vi "_power value.vi"(6 "label":T1, 8 "error in (no error)":errorcluster, 10 "B":refnum<class "Value.lvclass">, 11 "A":refnum<class "Value.lvclass">) -> (0 "error out":errorcluster, 2 "C":refnum<class "Value.lvclass">, 3 "A out":refnum<class "Value.lvclass">)   [LabVIEW 2023, in "LabGRAD.lvlib" / "Value.lvclass"]
uses:
  Value.lvclass
  UiObjects/string control.ctl
  operation.ctl
  Value.lvclass/Value.ctl
  UiObjects/UiObjects.lvclass
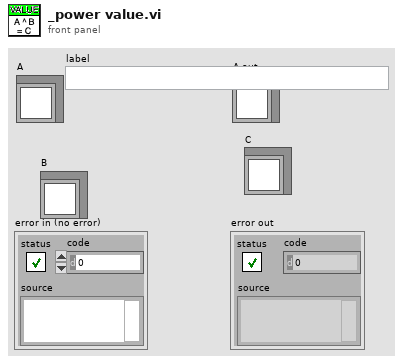
[diagram p1: front panel]
types:
  T1 = typedef "UiObjects.lvlib/UiObjects.lvclass/string control.ctl" = string
  T2 = typedef "LabGRAD.lvlib/Value.lvclass/operation.ctl" = enum16{"nop", "add", "subtract", "power", "multiply", "divide", "tanh"}
  T3 = typedef "UiObjects.lvlib/UiObjects.lvclass/numeric value control.ctl" = dbl
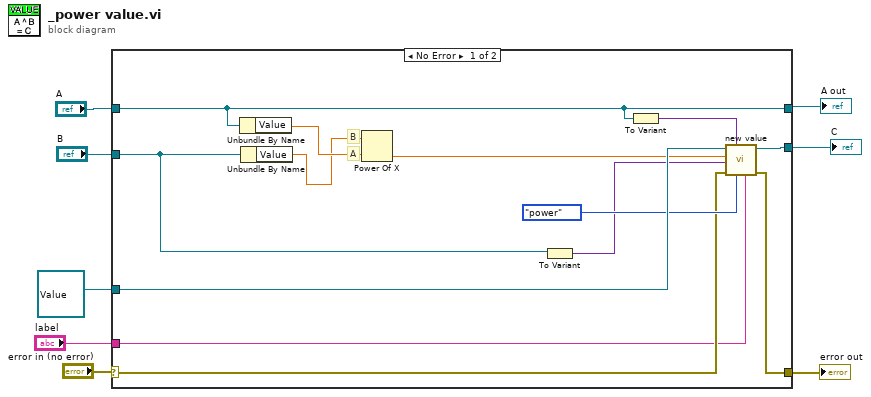
[diagram p0: block diagram]
diagram:
  n1 = case shown="No Error" "error in (no error)" {
    selector: "error in (no error)" -> [w11 w24]
    tunnel: [w10 w24] -> w6
    tunnel: [w21 w23] -> w7
    tunnel: "A" -> [w21 w23]
    tunnel: [w18 w22] -> w3
    tunnel: refnum<class "Value.lvclass"> refnum ("B") -> [w17 w22]
    tunnel: "B" -> [w14 _]
    tunnel: "label" -> [w9 _]
    frame No Error {
      # "A"
      # "B"
      n2 = Unbundle By Name(w21) -> ("Value"=w20:T3)
      n3 = Unbundle By Name(w14) -> ("Value"=w19:T3)
      n4 = Power Of X(1:w20, 2:w19) -> (0:w15:T3)
      n5 = To Variant(anything=w14) -> (Variant=w12:variant)
      n6 = To Variant(anything=w21) -> (Variant=w16:variant)
      n7 = call "new value.vi"("Label"=w9, "operation"=operation."power", "Previous"=w16, "error in (no error)"=w11, "Other"=w12, "data"=w15, "Value in"=w17) -> ("error out"=w10:errorcluster, "Value out"=w18:refnum<class "Value.lvclass">)  [unwired: 3 in]
    }
    frame Error {
    }
  }
  "error out" <- w6
  "A out" <- w7
  "C" <- w3
